vi "Diff_Drive_System_Act.vi"(6 "FPGA_Time_Seconds":dbl, 9 "Right Speed":dbl, 10 "Left Speed":dbl, 11 "Diff_Drive_Device_Refs":T1 {"GyroDevRef"."Sample Rate" min=0.25 max=100.0 step=0.25}) -> ()   [LabVIEW 2019]
uses:
  Diff_Drive_System_Device_Refs.ctl
  <vilib>/Rock Robotics/WPI/Gyro/WPI_GyroDevRef.ctl
  <vilib>/Rock Robotics/SystemInterfaces/AI/FPGA_AIChannel.ctl
  <vilib>/Rock Robotics/SystemInterfaces/spilib/spi_bus.ctl
  <vilib>/Rock Robotics/WPI/RobotDrive/WPI_RobotDriveDevRef.ctl
  <vilib>/Rock Robotics/WPI/MotorControl/WPI_MotorControlDeviceRef.ctl
  <vilib>/Rock Robotics/WPI/MotorControl/WPI_MotorControlType.ctl
  <vilib>/Rock Robotics/SystemInterfaces/DIO/FPGA_DIOPWMChannel.ctl
  <vilib>/Rock Robotics/WPI/PWM/WPI_PWMDeadband.ctl
  <vilib>/Rock Robotics/SystemInterfaces/DIO/FPGA_DIOChannel.ctl
  <vilib>/Rock Robotics/WPI/Encoder/WPI_EncoderDevRef.ctl
  <vilib>/Rock Robotics/SystemInterfaces/Encoder/FPGA_EncoderIdx.ctl
  <vilib>/Rock Robotics/SystemInterfaces/Counter/FPGA_CounterCtrSystemIndex.ctl
  <vilib>/Rock Robotics/WPI/Encoder/WPI_EncoderType.ctl
  <vilib>/Rock Robotics/WPI/ThirdParty/JAS_Junk/TrajLib/SlewRateLimiter_New.vi
  <vilib>/Rock Robotics/WPI/ThirdParty/JAS_Junk/TrajLib/SlewRateLimiter_Reset.vi
  <vilib>/Rock Robotics/WPI/ThirdParty/JAS_Junk/TrajLib/SlewRateLimiter_Calculate.vi
  <vilib>/Rock Robotics/WPI/ThirdParty/JAS_Junk/TrajLib/SlewRateLimiter_SetRate.vi
  <vilib>/Rock Robotics/WPI/ThirdParty/JAS_Junk/TrajLib/SimpleMotorFF_Calculate.vi
  <vilib>/Rock Robotics/WPI/ThirdParty/JAS_Junk/TrajLib/PIDController_AtSetpoint.vi
  <vilib>/Rock Robotics/WPI/ThirdParty/JAS_Junk/TrajLib/PIDController_SetPIDF.vi
  <vilib>/Rock Robotics/WPI/ThirdParty/JAS_Junk/TrajLib/PIDController_SetDerivativeFilter.vi
  <vilib>/Rock Robotics/WPI/ThirdParty/JAS_Junk/TrajLib/PIDController_SetIntegratorRange.vi
  <vilib>/Rock Robotics/WPI/ThirdParty/JAS_Junk/TrajLib/PIDController_SetTolerancePandV.vi
  <vilib>/Rock Robotics/WPI/ThirdParty/JAS_Junk/TrajLib/PIDController_DisableContinousInput.vi
  <vilib>/Rock Robotics/WPI/ThirdParty/JAS_Junk/TrajLib/PIDController_EnableContinousInput.vi
  <vilib>/Rock Robotics/WPI/ThirdParty/JAS_Junk/TrajLib/PIDController_Reset.vi
  <vilib>/Rock Robotics/WPI/ThirdParty/JAS_Junk/TrajLib/PIDController_New.vi
  <vilib>/Rock Robotics/WPI/ThirdParty/JAS_Junk/TrajLib/PIDController_SetOutputLimits.vi
  <vilib>/Rock Robotics/WPI/ThirdParty/JAS_Junk/TrajLib/PIDController_NewPeriod.vi
  <vilib>/Rock Robotics/SystemInterfaces/NetworkCommunication/NetComm_UsageReport_report.vi
  Diff_Drive_System_Globals.vi
  <vilib>/Rock Robotics/WPI/ThirdParty/JAS_Junk/TrajLib/Util_LibraryGlobals.vi
  <vilib>/Rock Robotics/WPI/ThirdParty/JAS_Junk/TrajLib/PIDController_AdvCalculate_FF_Sp_Pv.vi
  <vilib>/Rock Robotics/WPI/ThirdParty/JAS_Junk/TrajLib/Trajectory_Library.lvlib
panel:
  # "Analog"
  # "XRS"
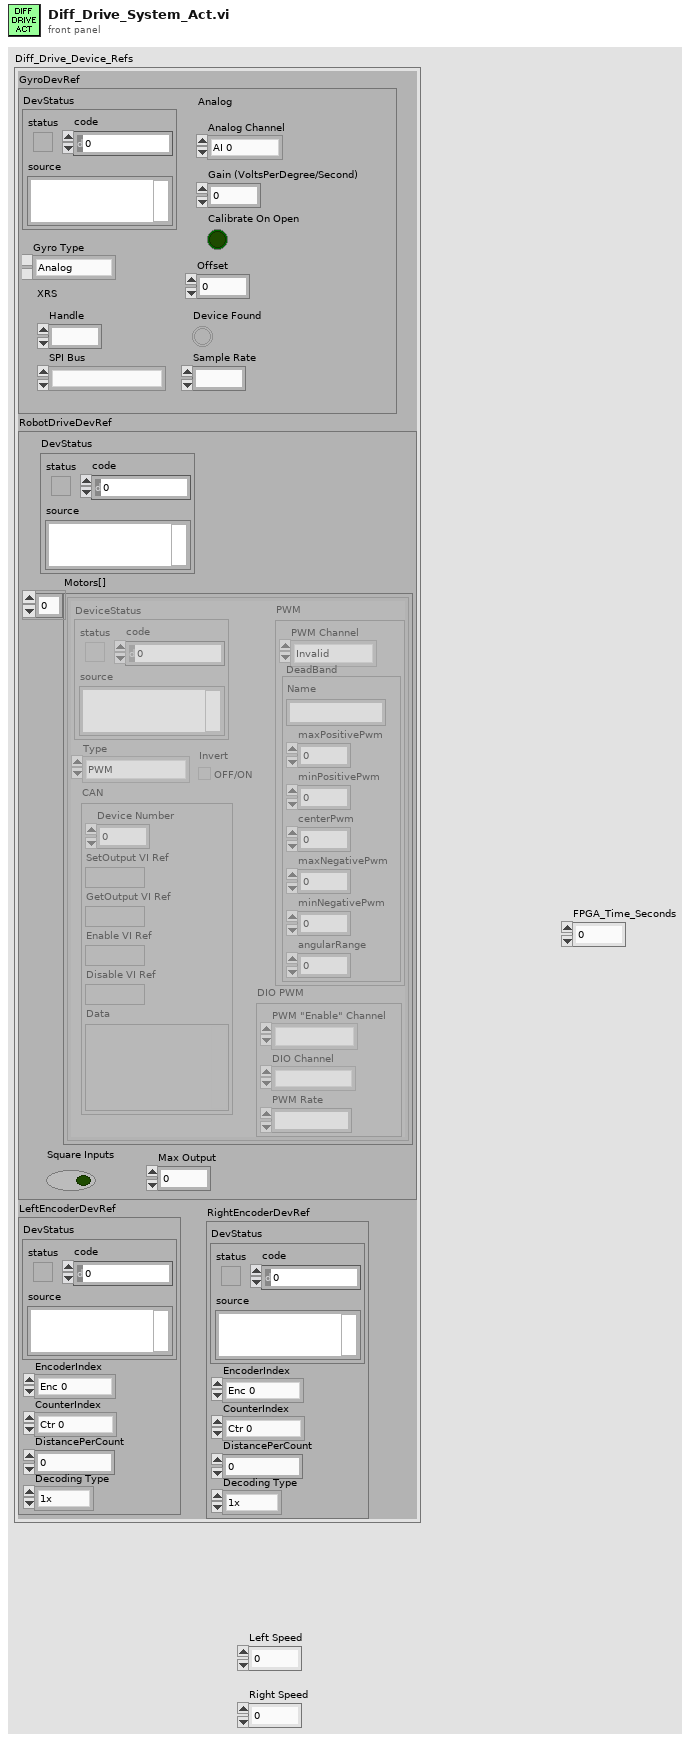
[diagram p1: front panel]
types:
  T1 = typedef "Diff_Drive_System_Device_Refs.ctl" = cluster{"GyroDevRef":T2, "RobotDriveDevRef":T5, "LeftEncoderDevRef":T11, "RightEncoderDevRef":T11}
  T2 = typedef "WPI_GyroDevRef.ctl" = cluster{"DevStatus":errorcluster, "Analog Channel":T3, "Gain (VoltsPerDegree/Second)":dbl, "Gyro Type":enum16{"Analog", "XRS450"}, "Handle":i32, "SPI Bus":T4, "Device Found":bool, "Sample Rate":dbl, "Calibrate On Open":bool, "Offset":dbl}
  T3 = typedef "FPGA_AIChannel.ctl" = enum8{"AI 0", "AI 1", "AI 2", "AI 3", "AI MXP 0", "AI MXP 1", "AI MXP 2", "AI MXP 3", "Invalid"}
  T4 = typedef "spi_bus.ctl" = enum16{"SPI On-Board, CS0", "SPI On-Board, CS1", "SPI On-Board, CS2", "SPI On-Board, CS3", "SPI MXP", "Invalid"}
  T5 = typedef "WPI_RobotDriveDevRef.ctl" = cluster{"DevStatus":errorcluster, "Motors[]":T6[], "Square Inputs":bool, "Max Output":dbl}
  T6 = typedef "WPI_MotorControlDeviceRef.ctl" = cluster{"DeviceStatus":errorcluster, "Type":T7, "PWM":cluster{"PWM Channel":T8, "DeadBand":T9}, "CAN":cluster{"Device Number":u8, "SetOutput VI Ref":variant, "GetOutput VI Ref":variant, "Enable VI Ref":variant, "Disable VI Ref":variant, "Data":variant}, "Invert":bool, "DIO PWM":cluster{"PWM \"Enable\" Channel":T8, "DIOChannel":T10, "PWM Rate":dbl}}
  T7 = typedef "WPI_MotorControlType.ctl" = enum16{"PWM", "CAN", "DIO PWM"}
  T8 = typedef "FPGA_DIOPWMChannel.ctl" = enum8{"PWM 0", "PWM 1", "PWM 2", "PWM 3", "PWM 4", "PWM 5", "PWM 6", "PWM 7", "PWM 8", "PWM 9", "PWM MXP 0", "PWM MXP 1", "PWM MXP 2", "PWM MXP 3", "PWM MXP 4", "PWM MXP 5", "PWM MXP 6", "PWM MXP 7", "PWM MXP 8", "PWM MXP 9", "Invalid"}
  T9 = typedef "WPI_PWMDeadband.ctl" = cluster{"Name":string, "maxPositivePwm":i32, "minPositivePwm":i32, "centerPwm":i32, "maxNegativePwm":i32, "minNegativePwm":i32, "angularRange":u16}
  T10 = typedef "FPGA_DIOChannel.ctl" = enum8{"DIO 0", "DIO 1", "DIO 2", "DIO 3", "DIO 4", "DIO 5", "DIO 6", "DIO 7", "DIO 8", "DIO 9", "DIO MXP 0", "DIO MXP 1", "DIO MXP 2", "DIO MXP 3", "DIO MXP 4", "DIO MXP 5", "DIO MXP 6", "DIO MXP 7", "DIO MXP 8", "DIO MXP 9", "DIO MXP 10", "DIO MXP 11", "DIO MXP 12", "DIO MXP 13", "DIO MXP 14", "DIO MXP 15", "SPI Port CS1", "SPI Port CS2", "SPI Port CS3", "SPI Port MISO", "SPI Port MOSI", "Invalid"}
  T11 = typedef "WPI_EncoderDevRef.ctl" = cluster{"DevStatus":errorcluster, "EncoderIndex":T12, "CounterIndex":T13, "DistancePerCount":dbl, "Decoding Type":T14}
  T12 = typedef "FPGA_EncoderIdx.ctl" = enum8{"Enc 0", "Enc 1", "Enc 2", "Enc 3", "Enc 4", "Enc 5", "Enc 6", "Enc 7", "Invalid"}
  T13 = typedef "FPGA_CounterCtrSystemIndex.ctl" = enum8{"Ctr 0", "Ctr 1", "Ctr 2", "Ctr 3", "Ctr 4", "Ctr 5", "Ctr 6", "Ctr 7", "Invalid"}
  T14 = typedef "WPI_EncoderType.ctl" = enum16{"1x", "2x", "4x"}
  T15 = typedef "Trajectory_Library.lvlib/SIMPLE_MOTOR_FF.ctl" = cluster{"Ks":dbl, "Kv":dbl, "Ka":dbl, "KnInv":dbl}
  T16 = typedef "Trajectory_Library.lvlib/PID_ADV_LIMITS.ctl" = cluster{"MaxInput":dbl, "MinInput":dbl, "Continuous":bool, "MaxOutput":dbl, "MinOutput":dbl}
  T17 = typedef "Trajectory_Library.lvlib/PID_ADV_TUNING.ctl" = cluster{"Kf":dbl, "Kp":dbl, "Ki":dbl, "Kd":dbl, "MaximumIntegral":dbl, "MinimumIntegral":dbl, "Filter Derivative":bool}
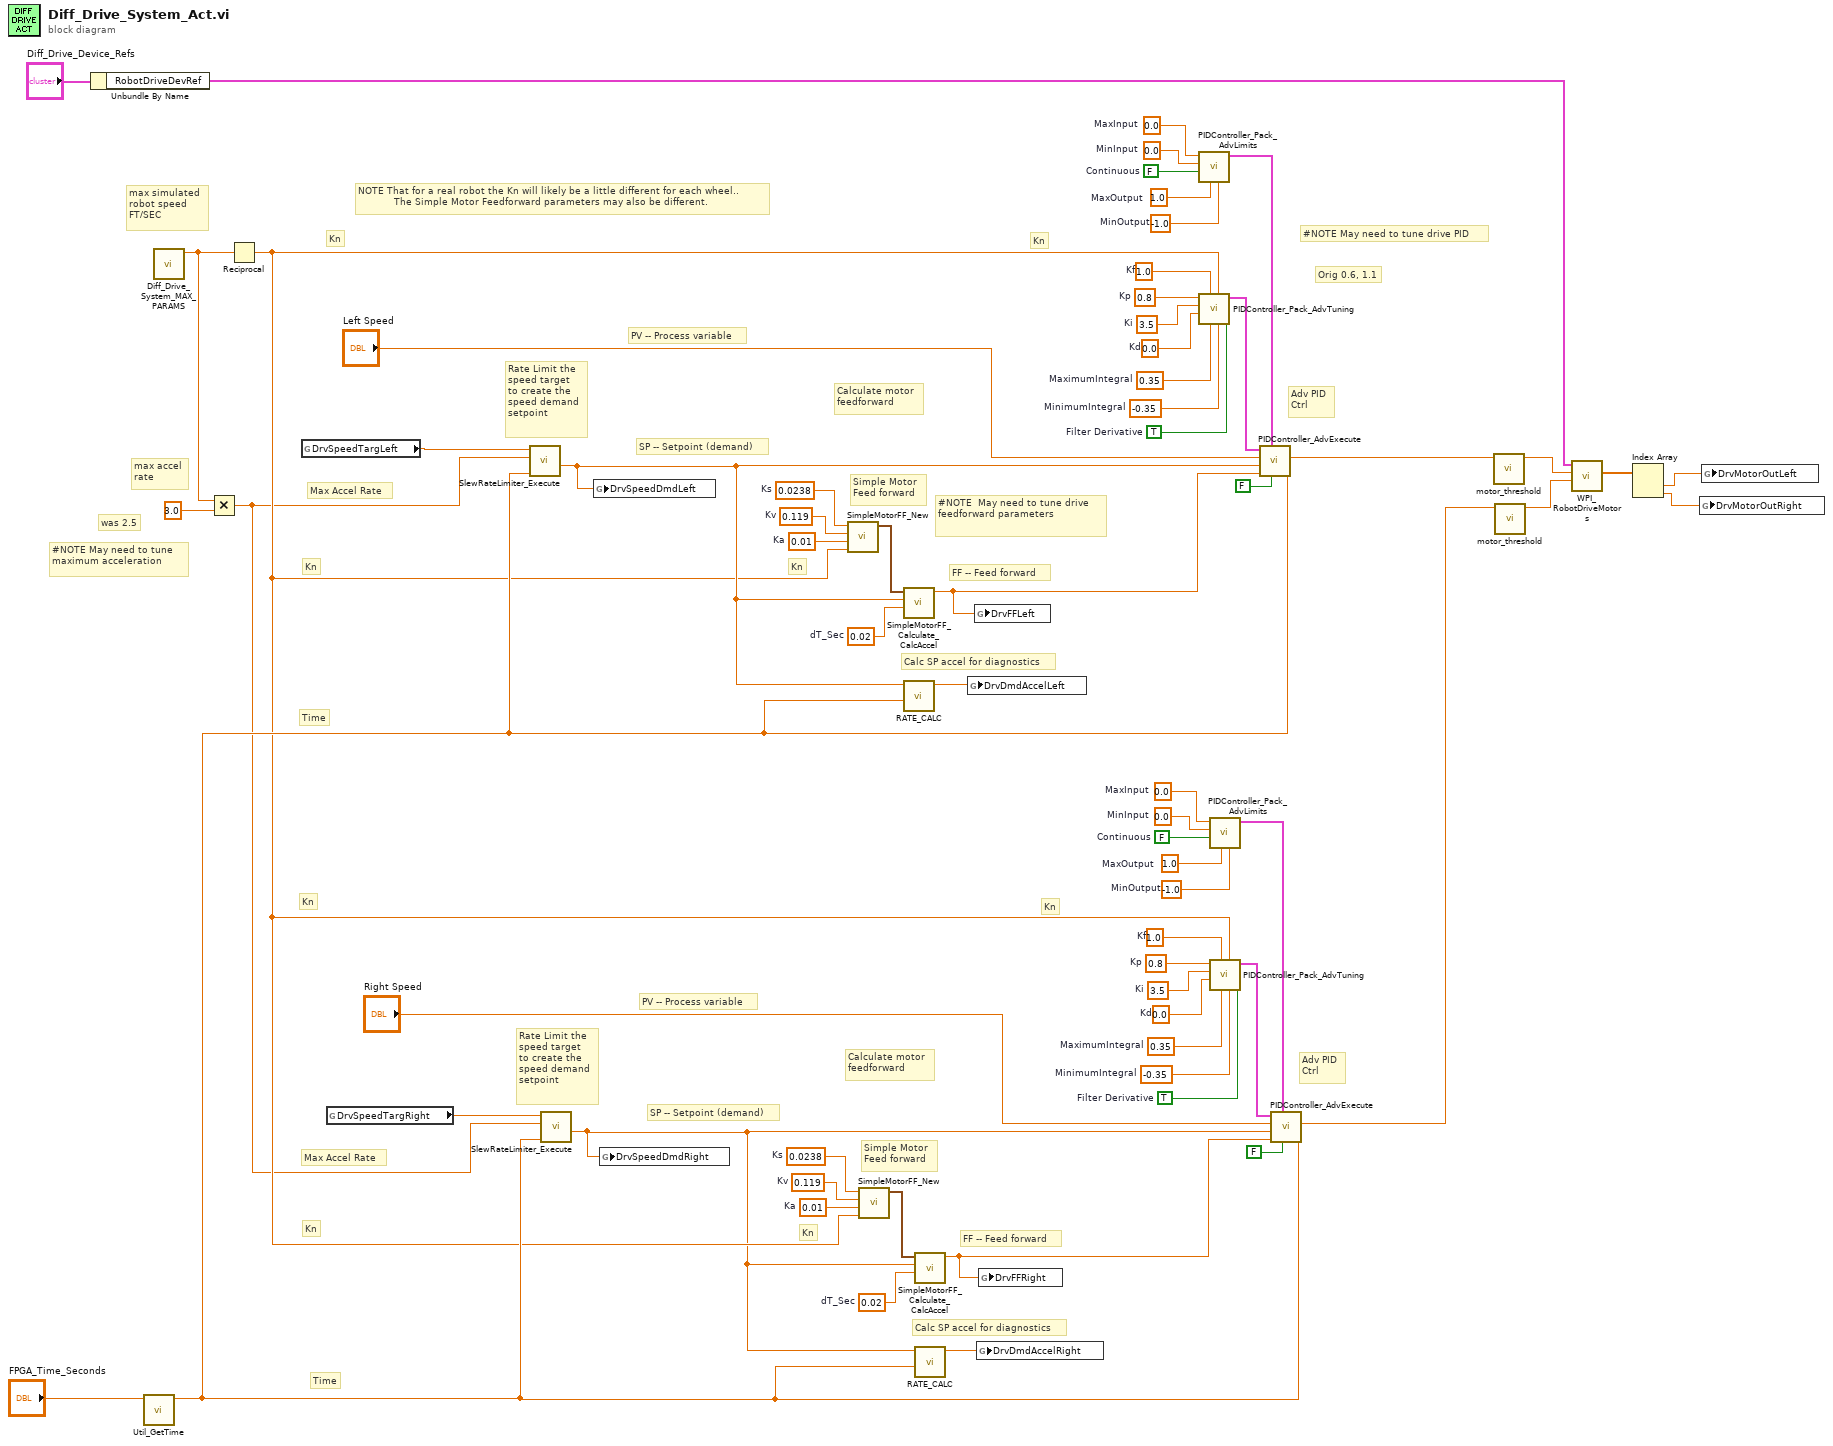
[diagram p0: block diagram]
diagram:
  w25 = 0.8  # Kp
  w24 = 3.5  # Ki
  w23 = 0.0  # Kd
  w22 = 1.0  # Kf
  w21 = 0.35  # MaximumIntegral
  w20 = -0.35  # MinimumIntegral
  w19 = TRUE  # Filter Derivative
  w17 = 0.0  # MinInput
  w16 = FALSE  # Continuous
  w15 = 1.0  # MaxOutput
  w18 = -1.0  # MinOutput
  w14 = 0.0  # MaxInput
  w30 = 0.02  # dT_Sec
  w28 = 0.0238  # Ks
  w27 = 0.119  # Kv
  w26 = 0.01  # Ka
  w50 = 0.8  # Kp
  w49 = 3.5  # Ki
  w48 = 0.0  # Kd
  w47 = 1.0  # Kf
  w46 = 0.35  # MaximumIntegral
  w45 = -0.35  # MinimumIntegral
  w44 = TRUE  # Filter Derivative
  w42 = 0.0  # MinInput
  w41 = FALSE  # Continuous
  w40 = 1.0  # MaxOutput
  w43 = -1.0  # MinOutput
  w39 = 0.0  # MaxInput
  w56 = 0.02  # dT_Sec
  w54 = 0.0238  # Ks
  w53 = 0.119  # Kv
  w52 = 0.01  # Ka
  # "Orig 0.6, 1.1"
  # "NOTE That for a real robot the Kn will likely be a little different for each wheel..\n            The Simple Motor Feedforward parameters may also be different."
  # "Max Accel Rate"
  # "Max Accel Rate"
  # "Time"
  # "Kn"
  # "Kn"
  # "Kn"
  # "Kn"
  # "Time"
  # "Kn"
  # "PV -- Process variable"
  # "Kn"
  # "Calc SP accel for diagnostics"
  # "FF -- Feed forward"
  # "SP -- Setpoint (demand)"
  # "Adv PID\nCtrl"
  # "Calculate motor\nfeedforward"
  # "Rate Limit the \nspeed target\nto create the\nspeed demand\nsetpoint"
  # "Simple Motor\nFeed forward"
  # "Kn"
  # "PV -- Process variable"
  # "Kn"
  # "Calc SP accel for diagnostics"
  # "FF -- Feed forward"
  # "SP -- Setpoint (demand)"
  # "Adv PID\nCtrl"
  # "Calculate motor\nfeedforward"
  # "was 2.5"
  # "Rate Limit the \nspeed target\nto create the\nspeed demand\nsetpoint"
  # "Simple Motor\nFeed forward"
  # "#NOTE May need to tune drive PID"
  # "#NOTE May need to tune maximum acceleration"
  # "#NOTE  May need to tune drive feedforward parameters"
  # "max simulated\nrobot speed\nFT/SEC"
  # "max accel\nrate"
  n1 = Unbundle By Name("Diff_Drive_Device_Refs") -> ("RobotDriveDevRef"=w59:T5)
  n2 = call <vilib>:"Util_GetTime.vi"("Pass_Through_Time"="FPGA_Time_Seconds") -> ("FPGA_Time_Seconds"=w10:dbl)  [unwired: 9 in, 1 out]
  n3 = call "Diff_Drive_System_MAX_PARAMS.vi"() -> ("Max Speed Ft/Sec"=w34:dbl)  [unwired: 10 in, 1 out]
  n4 = Multiply(x=w34, y=3.0 ("x")) -> (x*y=w8:dbl)
  n5 = Reciprocal(x=w34) -> (1/x=w9:dbl)
  n6 = global read "Diff_Drive_System_Globals.vi" "DrvSpeedTargLeft"() -> (w51:dbl)
  n7 = global read "Diff_Drive_System_Globals.vi" "DrvSpeedTargRight"() -> (w6:dbl)
  n8 = call <vilib>:"SlewRateLimiter_Execute.vi"("Time"=w10, "PositiveRate"=w8, "Input"=w51) -> ("Output"=w36:dbl)  [unwired: 7 in, 1 out]
  n9 = call <vilib>:"SlewRateLimiter_Execute.vi"("Time"=w10, "PositiveRate"=w8, "Input"=w6) -> ("Output"=w3:dbl)  [unwired: 7 in, 1 out]
  n10 = global write "Diff_Drive_System_Globals.vi" "DrvSpeedDmdLeft"(w36) -> ()
  n11 = global write "Diff_Drive_System_Globals.vi" "DrvSpeedDmdRight"(w3) -> ()
  n12 = call <vilib>:"SimpleMotorFF_New.vi"("Kn"=w9, "Ka"=w52, "Kv"=w53, "Ks"=w54) -> ("SIMPLE_MOTOR_FF"=w55:T15)  [unwired: 7 in]
  n13 = call <vilib>:"SimpleMotorFF_New.vi"("Kn"=w9, "Ka"=w26, "Kv"=w27, "Ks"=w28) -> ("SIMPLE_MOTOR_FF"=w29:T15)  [unwired: 7 in]
  n14 = call <vilib>:"SimpleMotorFF_Calculate_CalcAccel.vi"("dT_Sec"=w56, "VelSp"=w36, "SIMPLE_MOTOR_FF"=w55) -> ("FeedForward"=w33:dbl)  [unwired: 8 in]
  n15 = call "RATE_CALC.vi"("Time"=w10, "Input"=w36) -> ("Output"=w35:dbl)  [unwired: 9 in]
  n16 = call <vilib>:"SimpleMotorFF_Calculate_CalcAccel.vi"("dT_Sec"=w30, "VelSp"=w3, "SIMPLE_MOTOR_FF"=w29) -> ("FeedForward"=w5:dbl)  [unwired: 8 in]
  n17 = call "RATE_CALC.vi"("Time"=w10, "Input"=w3) -> ("Output"=w4:dbl)  [unwired: 9 in]
  n18 = global write "Diff_Drive_System_Globals.vi" "DrvDmdAccelLeft"(w35) -> ()
  n19 = global write "Diff_Drive_System_Globals.vi" "DrvFFLeft"(w33) -> ()
  n20 = global write "Diff_Drive_System_Globals.vi" "DrvDmdAccelRight"(w4) -> ()
  n21 = global write "Diff_Drive_System_Globals.vi" "DrvFFRight"(w5) -> ()
  n22 = call <vilib>:"PIDController_Pack_AdvLimits.vi"("MinOutput"=w43, "MaxOutput"=w40, "Continuous"=w41, "MinInput"=w42, "MaxInput"=w39) -> ("Adv PID Limits"=w37:T16)  [unwired: 6 in]
  n23 = call <vilib>:"PIDController_Pack_AdvTuning.vi"("Filter Derivative"=w44, "MinimumIntegral"=w45, "Kn"=w9, "MaximumIntegral"=w46, "Kf"=w47, "Kd"=w48, "Ki"=w49, "Kp"=w50) -> ("Adv PID Tuning"=w38:T17)  [unwired: 3 in]
  n24 = call <vilib>:"PIDController_Pack_AdvLimits.vi"("MinOutput"=w18, "MaxOutput"=w15, "Continuous"=w16, "MinInput"=w17, "MaxInput"=w14) -> ("Adv PID Limits"=w12:T16)  [unwired: 6 in]
  n25 = call <vilib>:"PIDController_Pack_AdvTuning.vi"("Filter Derivative"=w19, "MinimumIntegral"=w20, "Kn"=w9, "MaximumIntegral"=w21, "Kf"=w22, "Kd"=w23, "Ki"=w24, "Kp"=w25) -> ("Adv PID Tuning"=w13:T17)  [unwired: 3 in]
  n26 = call <vilib>:"PIDController_AdvExecute.vi"("Time"=w10, "Auto"=FALSE, "Adv PID Limits"=w37, "FF-FeedForward"=w33, "SP-SetPoint"=w36, "PV-Measurement"="Left Speed", "Adv PID Tuning"=w38) -> ("CO-ControlOutput"=w32:dbl)  [unwired: 2 in, 2 out]
  n27 = call <vilib>:"PIDController_AdvExecute.vi"("Time"=w10, "Auto"=FALSE, "Adv PID Limits"=w12, "FF-FeedForward"=w5, "SP-SetPoint"=w3, "PV-Measurement"="Right Speed", "Adv PID Tuning"=w13) -> ("CO-ControlOutput"=w11:dbl)  [unwired: 2 in, 2 out]
  n28 = call "motor_threshold.vi"("motor in"=w32) -> ("motor out"=w63:dbl)  [unwired: 10 in]
  n29 = call "motor_threshold.vi"("motor in"=w11) -> ("motor out"=w64:dbl)  [unwired: 10 in]
  n30 = call <vilib>:"WPI_RobotDriveMotors.vi"("RightSpeed"=w64, "LeftSpeed"=w63, "RobotDriveDevRef"=w59) -> ("Motor Values"=w62:dbl[])  [unwired: 6 in, 2 out]
  n31 = Index Array(array=w62) -> (element #1=w58:dbl, element #2=w57:dbl)  [unwired: 2 in]
  n32 = global write "Diff_Drive_System_Globals.vi" "DrvMotorOutRight"(w57) -> ()
  n33 = global write "Diff_Drive_System_Globals.vi" "DrvMotorOutLeft"(w58) -> ()
